vi "NI-Linux-RT-64 Library Path.vi"() -> (0 "Path":path=path "/usr/lib/libserenial.io-ase.so.1")   [LabVIEW 2020, in "ase.lvlib" / "ase.lvclass"]
doc: "Path to shared library on NI-Linux-RT 64 bit systems."
uses:
  ase.lvclass
  ase.lvclass/ase.ctl
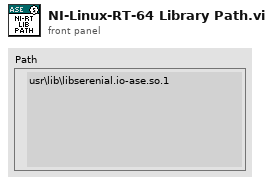
[diagram p1: front panel]
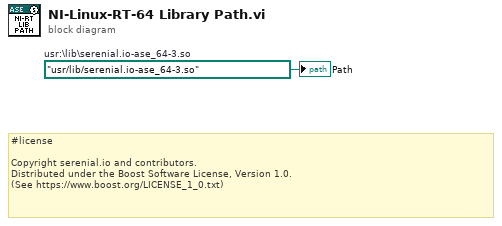
[diagram p0: block diagram]
diagram:
  w1 = path "/usr/lib/serenial.io-ase_64-3.so"  # usr:\lib\serenial.io-ase_64-3.so
  # "#license\n\nCopyright serenial.io and contributors.\nDistributed under the Boost Software License, Version 1.0.\n(See https://www.boost.org/LICENSE_1_0.txt)"
  "Path" <- w1
